vi "start_sweep.vi"(8 "error in (no error)":errorcluster, 11 "DL090503StimulatorScaffold in":refnum<class "StimulatorDL090503Scaffold.lvclass">) -> (0 "error out":errorcluster, 3 "DL090503StimulatorScaffold out":refnum<class "StimulatorDL090503Scaffold.lvclass">)   [LabVIEW 2010, in "StimulatorDL090503Scaffold.lvclass"]
uses:
  StimulatorDL090503Scaffold.lvclass
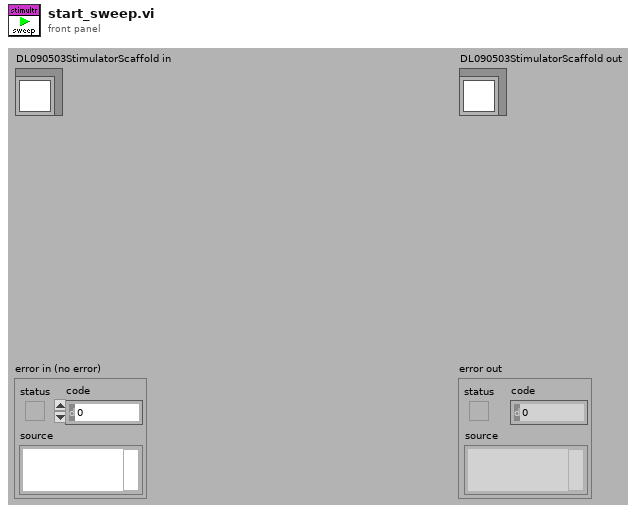
[diagram p1: front panel]
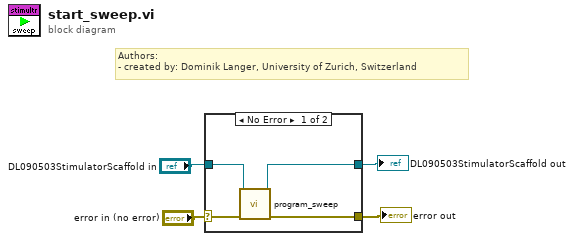
[diagram p0: block diagram]
diagram:
  # "Authors: \n- created by: Dominik Langer, University of Zurich, Switzerland"
  n1 = case shown="No Error" "error in (no error)" {
    selector: "error in (no error)" -> [w8 w10]
    tunnel: [w7 w10] -> w3
    tunnel: [w5 w9] -> w1
    tunnel: "DL090503StimulatorScaffold in" -> [w6 w9]
    frame No Error {
      n2 = call-dynamic "program_sweep.vi"("error in (no error)"=w8, "DL090503StimulatorScaffold in"=w6) -> ("error out"=w7:errorcluster, "DL090503StimulatorScaffold out"=w5:refnum<class "StimulatorDL090503Scaffold.lvclass">)  [unwired: 8 out]
    }
    frame Error {
    }
  }
  "error out" <- w3
  "DL090503StimulatorScaffold out" <- w1
